vi "Terminate.vi"(6 "Teller":refnum<class "Teller.lvclass">, 9 "Error":errorcluster, 10 "Actor":refnum<class "Actor.lvclass">, 11 "TEMPLATE Actor in":refnum<class "TEMPLATE Actor.lvclass">) -> (0 "Error out":errorcluster, 3 "TEMPLATE Actor out":refnum<class "TEMPLATE Actor.lvclass">)   [LabVIEW 2025, in "_Template.lvlib" / "Templates.lvlib" / "TEMPLATE Actor.lvlib" / "TEMPLATE Actor.lvclass"]
uses:
  TEMPLATE Actor.lvclass
  TEMPLATE Actor.lvclass/TEMPLATE Actor.ctl
  C:/git/jettl/src/jettl Tools/_Template/Templates/TEMPLATE Actor/TEMPLATE Actor/TEMPLATE Actor.lvclass
  C:/git/jettl/src/jettl/jettl/Actor/Actor/Actor.lvclass
  C:/git/jettl/src/jettl/jettl/Terminate Msg/Terminate/Terminate.lvclass
  jettl/jettl/Terminate Msg/Terminate Msg.lvlib
  jettl/jettl/Terminate Msg/Decorator.vi
  jettl/jettl/Actor/Actor/Actor.lvclass
  jettl/jettl/Teller/Teller/Teller.lvclass
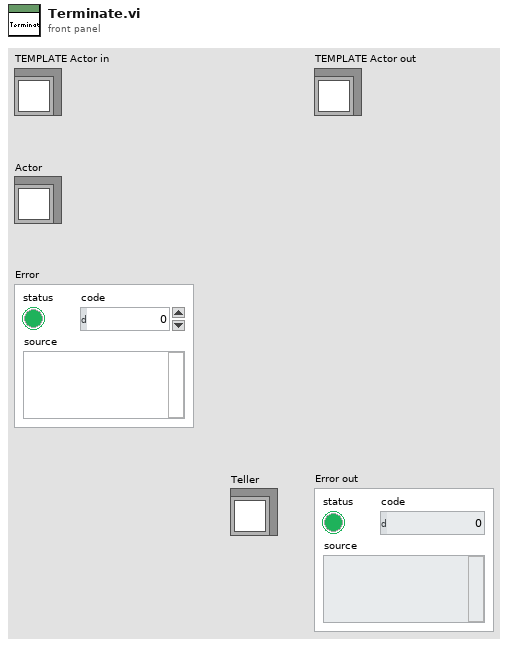
[diagram p1: front panel]
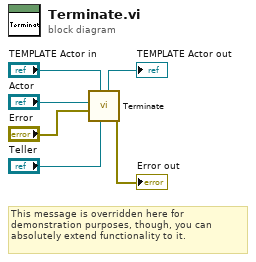
[diagram p0: block diagram]
diagram:
  # "This message is overridden here for demonstration purposes, though, you can absolutely extend functionality to it."
  n1 = call-poly "Terminate.vi"("Teller"="Teller", "Actor in"="TEMPLATE Actor in", "Error"="Error", "Actor"="Actor") -> ("Error out"=→"Error out":errorcluster, "Actor out"=→"TEMPLATE Actor out":refnum<class "TEMPLATE Actor.lvclass">)  [unwired: 6 in]
